vi "DAQ.Sampling.Configure.vi"(8 "error in (no error)":errorcluster, 11 "DAQmx in":refnum<class "DAQmx.lvclass">) -> (0 "error out":errorcluster, 2 "Restart Acquisition?":bool, 3 "DAQmx out":refnum<class "DAQmx.lvclass">)   [LabVIEW 2019, in "DAQmx.lvclass"]
uses:
  DAQmx.lvclass
  DAQmx.lvclass/DAQmx.ctl
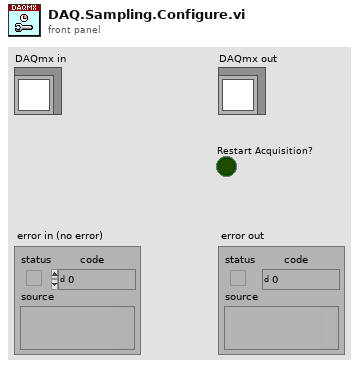
[diagram p1: front panel]
types:
  T1 = typedef "DAQmx.lvclass/DAQ.Config.Timing.Sampling--Cluster.ctl" = cluster{"Fs":dbl, "#s":i32}
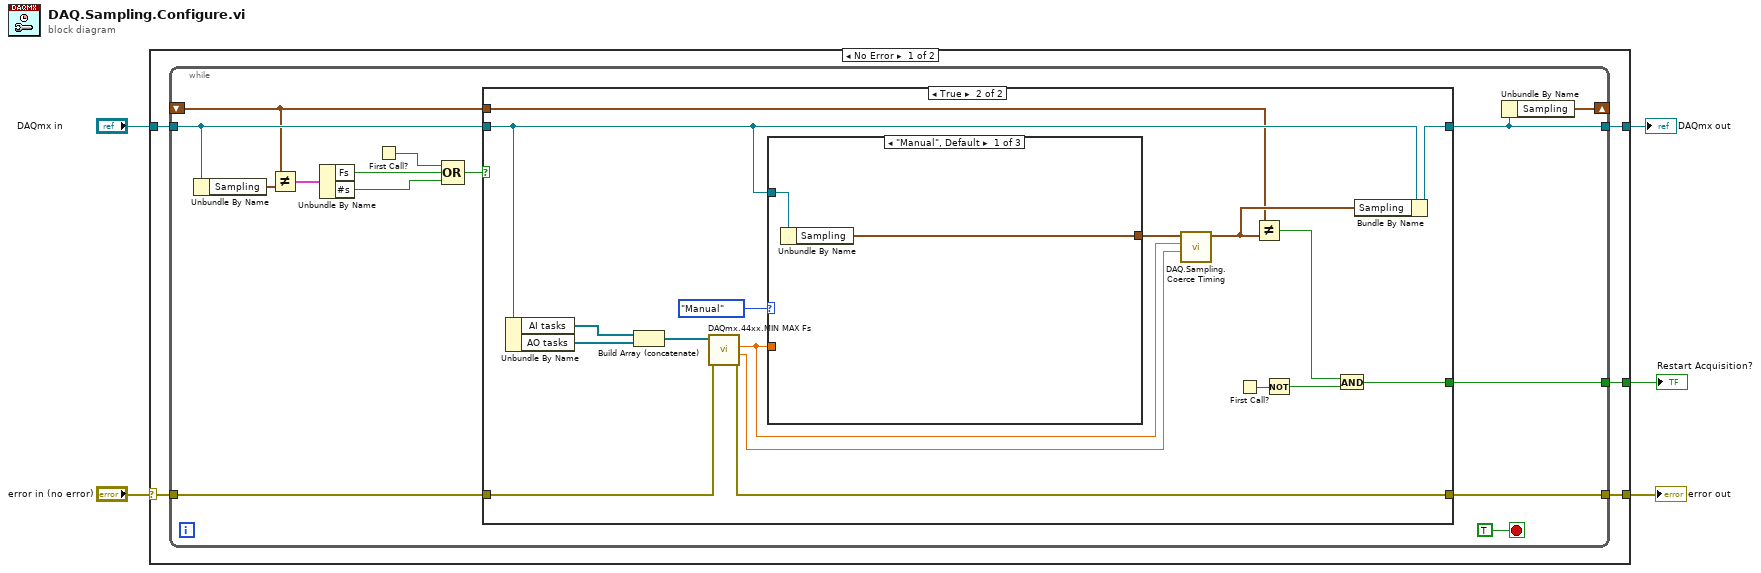
[diagram p0: block diagram]
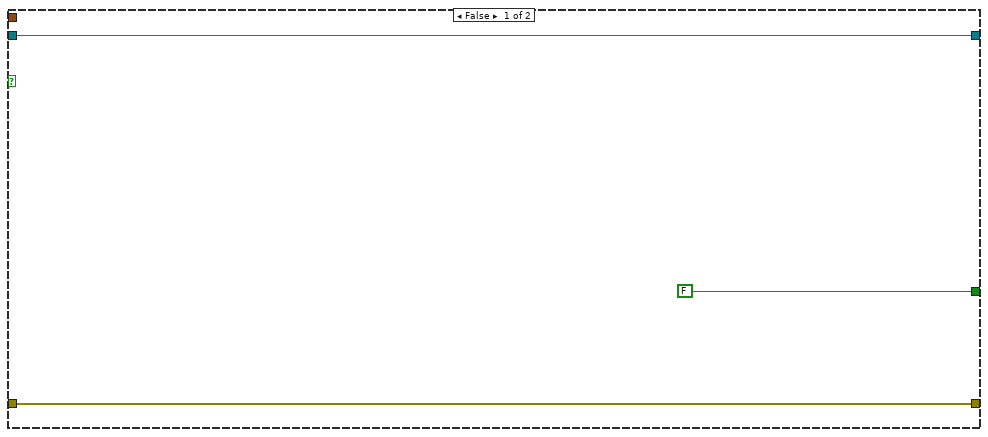
[diagram p2: hidden frame]
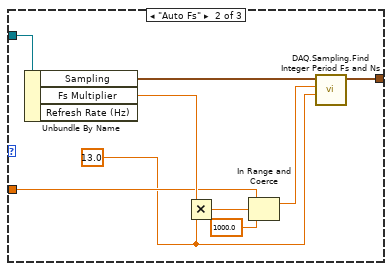
[diagram p3: hidden frame]
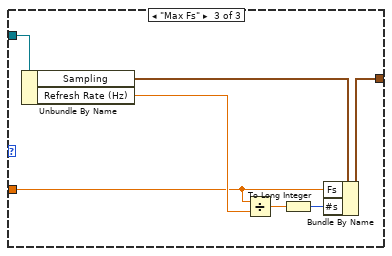
[diagram p4: hidden frame]
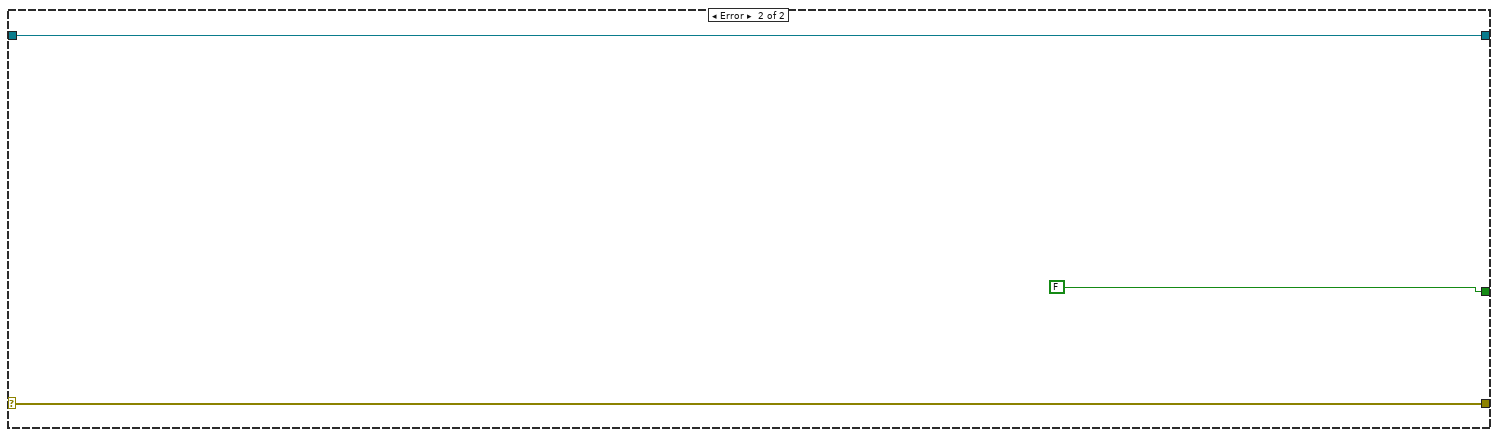
[diagram p5: hidden frame]
diagram:
  n1 = case shown="No Error" "error in (no error)" {
    selector: "error in (no error)" -> [w9 w65]
    tunnel: "DAQmx in" -> [w10 w64]
    tunnel: [w6 w64] -> w3
    tunnel: [w8 w65] -> w2
    tunnel: [w7 FALSE] -> w1
    frame No Error {
      n2 = while {
        tunnel: [w16] -> w7
        tunnel: w10 -> [w13]
        tunnel: [w14] -> w6
        tunnel: w9 -> [w22]
        tunnel: [w21] -> w8
        shift-right: [w23] -> _
        shift-left: _ -> [w12]
        stop <- TRUE stop-if-true
        n3 = Unbundle By Name(w13) -> ("Sampling"=w15:T1)
        n4 = Not Equal?(x=w12, y=w15) -> (x != y?=w11:cluster{"Fs":bool, "#s":bool})
        n5 = Unbundle By Name(w11) -> ("Fs"=w20:bool, "#s"=w19:bool)
        n6 = First Call?() -> (First Call?: T/F=w17:bool)
        n7 = Compound Arithmetic op=OR(w17, w20, w19) -> (w18:bool)
        n8 = case shown="True" w18 {
          tunnel: w22 -> [w27 w41]
          tunnel: [w27 w40] -> w21
          tunnel: [w26 w30] -> w14
          tunnel: w13 -> [w26 w31]
          tunnel: [FALSE w34] -> w16
          tunnel: w12 -> [_ w29]
          frame False {
          }
          frame True {
            n9 = Unbundle By Name(w31) -> ("AI tasks"=w33:refnum<k21>[], "AO tasks"=w32:refnum<k21>[])
            n10 = Build Array (concatenate)(w33, w32) -> (w44:refnum<k21>[])
            n11 = call "DAQmx.44xx.MIN MAX Fs.vi"("error in (no error)"=w41, "task []"=w44) -> ("error out"=w40:errorcluster, "Max(SampClk.MinRate) (S/s)"=w42:dbl, "Min(SampClk.MaxRate) (S/s)"=w39:dbl)  [unwired: 7 in]
            n12 = case shown="\"Manual\", Default" enum16{"Manual", "Auto Fs", "Max Fs"}."Manual" ("FsMode") {
              tunnel: w31 -> [w45 w50 w56]
              tunnel: w39 -> [_ w52 w59]
              tunnel: [w46 w49 w57] -> w43
              frame "Manual", Default {
                n13 = Unbundle By Name(w45) -> ("Sampling"=w46:T1)
              }
              frame "Auto Fs" {
                w47 = 13.0 ("y")
                n14 = Unbundle By Name(w50) -> ("Sampling"=w48:T1, "Fs Multiplier"=w53:dbl)  [unwired: 1 out]
                n15 = Multiply(x=w53, y=w47) -> (x*y=w55:dbl)
                n16 = In Range and Coerce(upper limit=w52, x=w55, lower limit=1000.0) -> (coerced(x)=w51:dbl)  [unwired: 1 out]
                n17 = call "DAQ.Sampling.Find Integer Period Fs and Ns.vi"("f in"=w47, "maxFs"=w51, "sampling in"=w48) -> ("sampling out"=w49:T1)  [unwired: 7 in, 1 out]
              }
              frame "Max Fs" {
                n18 = Unbundle By Name(w56) -> ("Sampling"=w58:T1, "Refresh Rate (Hz)"=w60:dbl)
                n19 = Divide(x=w59, y=w60) -> (x/y=w62:dbl)
                n20 = To Long Integer(number=w62) -> (32bit integer=w61:i32)
                n21 = Bundle By Name(cluster=w58, "Fs"=w59, "#s"=w61) -> (w57:T1)
              }
            }
            n22 = call "DAQ.Sampling.Coerce Timing.vi"("Min Fs"=w42, "Max Fs"=w39, "Sampling in"=w43) -> ("Sampling out"=w38:T1)  [unwired: 8 in]
            n23 = First Call?() -> (First Call?: T/F=w37:bool)
            n24 = Not Equal?(x=w29, y=w38) -> (x != y?=w35:bool)
            n25 = Not(x=w37) -> (.not. x?=w36:bool)
            n26 = And(x=w35, y=w36) -> (x .and. y?=w34:bool)
            n27 = Bundle By Name(cluster=w31, "Sampling"=w38) -> (w30:refnum<class "DAQmx.lvclass">)
          }
        }
        n28 = Unbundle By Name(w14) -> ("Sampling"=w23:T1)
      }
    }
    frame Error {
    }
  }
  "DAQmx out" <- w3
  "error out" <- w2
  "Restart Acquisition?" <- w1
